vi "readXMLFile.vi"(8 "error in (no error)":errorcluster, 10 "Path":path, 11 "SettingsManager in":refnum<class "SettingsManager.lvclass">) -> (0 "error out":errorcluster, 3 "SettingsManager out":refnum<class "SettingsManager.lvclass">)   [LabVIEW 2009, in "Tools.lvlib" / "Settings.lvlib" / "SettingsManager.lvclass"]
uses:
  SettingsManager.lvclass
  XmlParser.lvclass
  SettingsManager.lvclass/SettingsManager.ctl
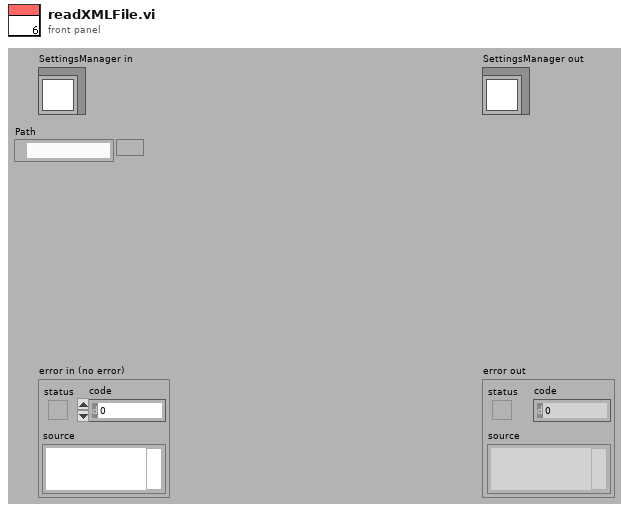
[diagram p1: front panel]
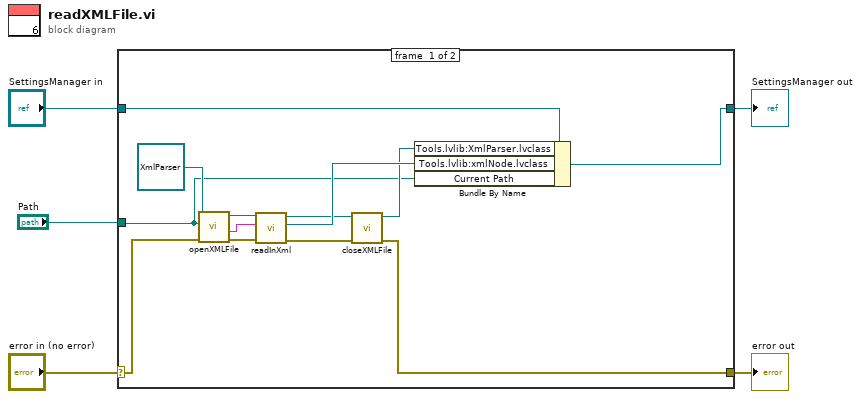
[diagram p0: block diagram]
diagram:
  n1 = case shown="No Error" "error in (no error)" {
    selector: "error in (no error)" -> [w17 w20]
    tunnel: [w8 w20] -> w4
    tunnel: [w15 w19] -> w2
    tunnel: "SettingsManager in" -> [w16 w19]
    tunnel: "Path" -> [w6 _]
    frame #0 {
      n2 = call "openXMLFile.vi"("error in (no error)"=w17, "Path"=w6, "XmlParser in"=refnum<class "XmlParser.lvclass"> refnum ("Tools.lvlib:XmlParser.lvclass")) -> ("error out"=w13:errorcluster, "xmlFileInput"=w12:string, "XmlParser out"=w14:refnum<class "XmlParser.lvclass">)  [unwired: 6 in]
      n3 = call "readInXml.vi"("error in (no error)"=w13, "xmlString"=w12, "XmlParser in"=w14) -> ("error out"=w9:errorcluster, "xmlNode"=w11:refnum<class "xmlNode.lvclass">, "XmlParser out"=w10:refnum<class "XmlParser.lvclass">)  [unwired: 6 in]
      n4 = call-dynamic "closeXMLFile.vi"("error in (no error)"=w9, "XmlParser in"=w10) -> ("error out"=w8:errorcluster, "XmlParser out"=w7:refnum<class "XmlParser.lvclass">)  [unwired: 8 in]
      n5 = Bundle By Name(cluster=w16, "Tools.lvlib:XmlParser.lvclass"=w7, "Tools.lvlib:xmlNode.lvclass"=w11, "Current Path"=w6) -> (w15:refnum<class "SettingsManager.lvclass">)
    }
    frame #1 {
    }
  }
  "error out" <- w4
  "SettingsManager out" <- w2
